vi "Required Buffer Sizes.vi"(8 "error in (no error)":errorcluster, 11 "Group Configuration in":refnum<class "Group Configuration.lvclass">) -> (0 "error out":errorcluster, 1 "string size":u64 format="%d bytes", 2 "engine size":u64 format="%d bytes", 3 "Group Configuration out":refnum<class "Group Configuration.lvclass">)   [LabVIEW 2019, in "DSF Core.lvlib" / "Group Configuration.lvclass"]
uses:
  Group Configuration.lvclass
  Group Configuration.lvclass/Group Configuration.ctl
  Transfer/Transfer Configuration.lvclass
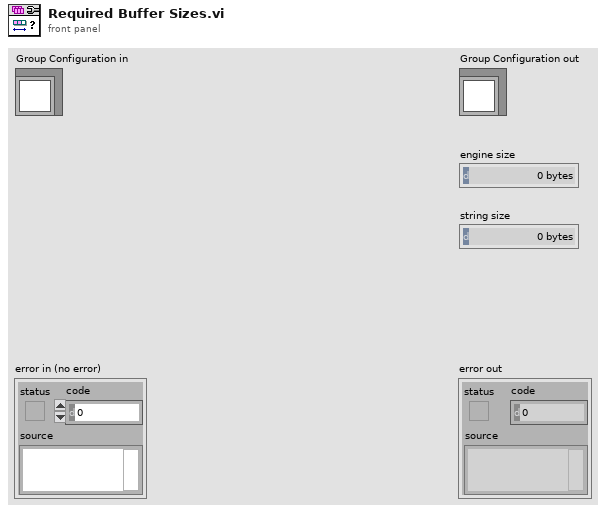
[diagram p1: front panel]
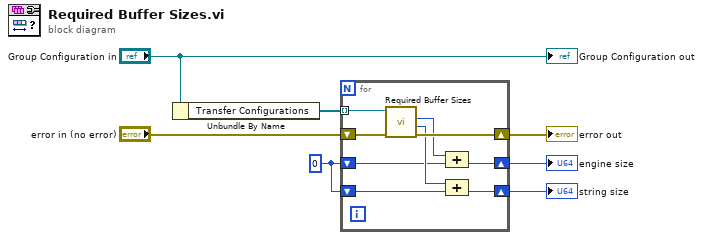
[diagram p0: block diagram]
diagram:
  w3 = u64 0 ("string size")
  n1 = Unbundle By Name("Group Configuration in") -> ("Transfer Configurations"=w5:refnum<class "Transfer Configuration.lvclass">[])
  n2 = for {
    shift-right: [w16] -> w7
    shift-left: "error in (no error)" -> [w15]
    tunnel: w5 -> [w14] mode=indexing
    shift-right: [w10] -> w2
    shift-left: w3 -> [w11]
    shift-right: [w13] -> w1
    shift-left: w3 -> [w9]
    n3 = call-dynamic "Required Buffer Sizes.vi"("error in (no error)"=w15, "Transfer Configuration in"=w14) -> ("error out"=w16:errorcluster, "string size"=w12:u64, "engine size"=w8:u64)  [unwired: 6 in, 1 out]
    n4 = Compound Arithmetic op=ADD(w8, w11) -> (w10:u64)
    n5 = Compound Arithmetic op=ADD(w12, w9) -> (w13:u64)
  }
  "error out" <- w7
  "string size" <- w1
  "engine size" <- w2
  "Group Configuration out" <- "Group Configuration in"
